vi "Version Updates.vi"(6 "Build Spec":string, 8 "error in (no error)":errorcluster, 9 "Target":string, 10 "Project":path, 11 "Option Set in":refnum<class "Option Set.lvclass">) -> (0 "error out":errorcluster)   [LabVIEW 2014, in "G CLI LvBuild.lvlib"]
uses:
  G CLI LvBuild.lvlib
  <vilib>/Wiresmith Technology/G CLI/Argument Parser/Option Set Class/Option Set.lvclass
  <vilib>/AppBuilder/AB_API_Simple/Build Specification Version.ctl
  <vilib>/AppBuilder/AB_API_Simple/Set Build Specification Version (path).vi
  <vilib>/AppBuilder/AB_API_Simple/Get Build Specification Version (path).vi
  <vilib>/AppBuilder/AB_API_Simple/NI_App_Builder_API.lvlib
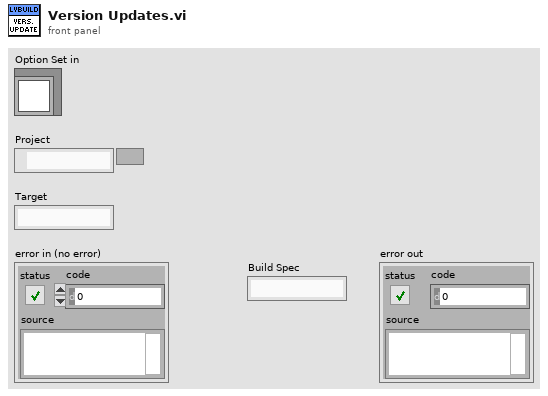
[diagram p1: front panel]
types:
  T1 = typedef "NI_App_Builder_API.lvlib/Build Specification Version.ctl" = cluster{"Major":u16, "Minor":u16, "Fix":u16, "Build":u16}
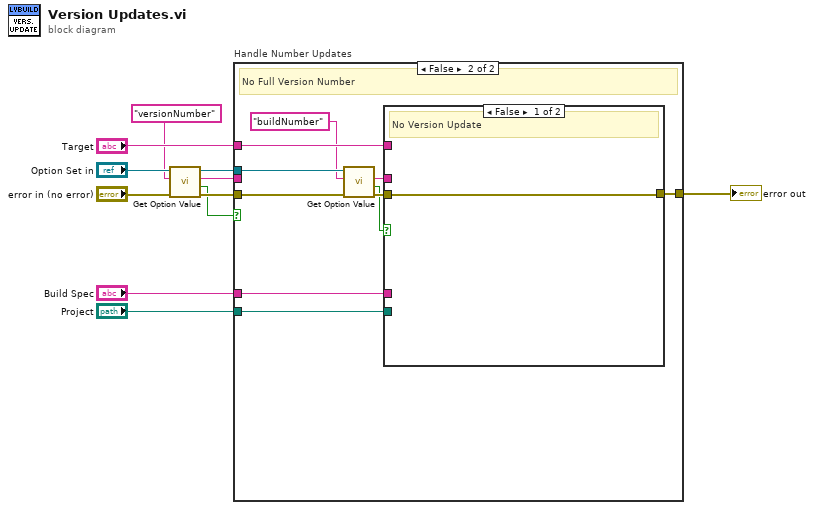
[diagram p0: block diagram]
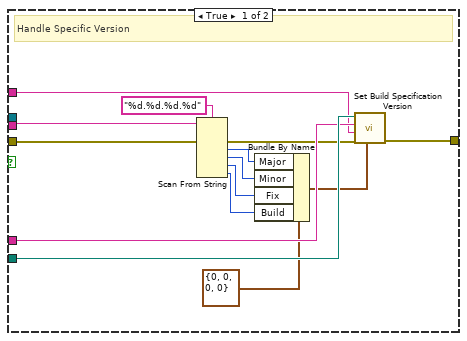
[diagram p2: hidden frame]
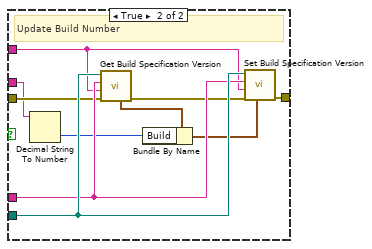
[diagram p3: hidden frame]
diagram:
  n1 = call <vilib>:"Get Option Value.vi"("error in (no error)"="error in (no error)", "Option Key"="versionNumber", "Option Set in"="Option Set in") -> ("error out"=w3:errorcluster, "Set"=w2:bool, "Value"=w4:string, "Option Set out"=w10:refnum<class "Option Set.lvclass">)  [unwired: 5 in]
  n2 = case "Handle Number Updates" shown="False" w2 {
    tunnel: w3 -> [w25 w34]
    tunnel: w4 -> [w20 _]
    tunnel: "Project" -> [w24 w33]
    tunnel: "Build Spec" -> [w23 w32]
    tunnel: "Target" -> [w22 w31]
    tunnel: [w12 w35] -> w11
    tunnel: w10 -> [_ w29]
    frame True {
      # "Handle Specific Version"
      n3 = Scan From String(format string="%d.%d.%d.%d", input string=w20, error in=w25) -> (error out=w21:errorcluster, output 1=w16:i32, output 2=w15:i32, output 3=w14:i32, output 4=w13:i32)  [unwired: 5 in, 2 out]
      n4 = Bundle By Name(cluster=T1 {"Major"=0, "Minor"=0, "Fix"=0, "Build"=0} ("Build Specification Version"), "Major"=w16, "Minor"=w15, "Fix"=w14, "Build"=w13) -> (w17:T1)
      n5 = call-poly <vilib>:"Set Build Specification Version.vi"("Build Specification Version"=w17, "error in (no error)"=w21, "Name of target (My Computer)"=w22, "Name of build specification"=w23, "Path to project"=w24) -> ("error out"=w12:errorcluster)  [unwired: 6 in]
    }
    frame False {
      # "No Full Version Number"
      n6 = call <vilib>:"Get Option Value.vi"("error in (no error)"=w34, "Option Key"="buildNumber", "Option Set in"=w29) -> ("error out"=w30:errorcluster, "Set"=w26:bool, "Value"=w27:string)  [unwired: 5 in, 1 out]
      n7 = case shown="False" w26 {
        tunnel: [w36 w46] -> w35
        tunnel: w33 -> [_ w45]
        tunnel: w32 -> [_ w44]
        tunnel: w31 -> [_ w43]
        tunnel: w30 -> [w36 w38]
        tunnel: w27 -> [_ w37]
        frame False {
          # "No Version Update"
        }
        frame True {
          # "Update Build Number"
          n8 = Decimal String To Number(string=w37) -> (number=w39:i32)  [unwired: 2 in, 1 out]
          n9 = call-poly <vilib>:"Get Build Specification Version.vi"("error in (no error)"=w38, "Name of target (My Computer)"=w43, "Name of build specification"=w44, "Path to project"=w45) -> ("error out"=w42:errorcluster, "Build Specification Version"=w41:T1)  [unwired: 6 in]
          n10 = Bundle By Name(cluster=w41, "Build"=w39) -> (w40:T1)
          n11 = call-poly <vilib>:"Set Build Specification Version.vi"("Build Specification Version"=w40, "error in (no error)"=w42, "Name of target (My Computer)"=w43, "Name of build specification"=w44, "Path to project"=w45) -> ("error out"=w46:errorcluster)  [unwired: 6 in]
        }
      }
    }
  }
  "error out" <- w11
